vi "Write_Accelerometer_To_Read.vi"(8 "error in (no error)":errorcluster, 9 "Read ERD List":T2[](array[typedef]) {"ERD Number" format="%.0x"}, 10 "GEA Inputs":T1 {"Destination" format="%.0x"; "Source" format="%.0x"}, 11 ".NET Refnum in":refnum<k24>) -> (0 "error out":errorcluster, 3 ".NET Refnum out":refnum<k24>)   [LabVIEW 2016]
doc: "This VI checks to see if Accelerometer ERD is in Read ERD List. If so it write to Accelerometer ERD. Writing toi this ERD updates ERD with latest Accelerometer data, which allows it to be read back from ERD."
uses:
  Common/LabVIEW GEA2 Toolkit/LabVIEW_GEA2_Toolkit.lvlibp/type defs/ERD Read Data In.ctl
  Common/LabVIEW GEA2 Toolkit/LabVIEW_GEA2_Toolkit.lvlibp/type defs/Data Type.ctl
  Common/LabVIEW GEA2 Toolkit/LabVIEW_GEA2_Toolkit.lvlibp/type defs/Source_Destination.ctl
  C:/Automation/DLLs/PC Dot Net/GeaCommunication.dll
  Common/LabVIEW GEA2 Toolkit/LabVIEW_GEA2_Toolkit.lvlibp/type defs/ERD Write Data In.ctl
  Common/LabVIEW GEA2 Toolkit/LabVIEW_GEA2_Toolkit.lvlibp
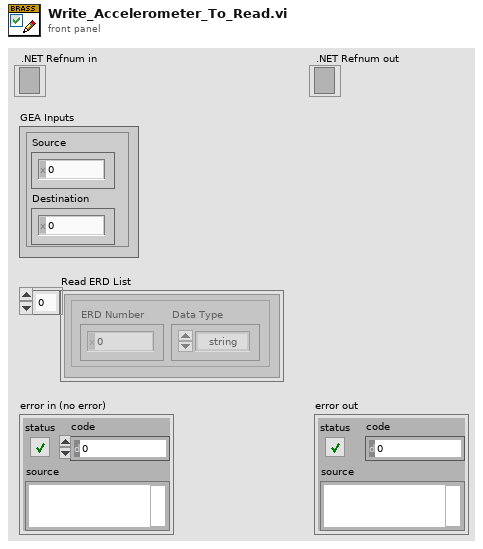
[diagram p1: front panel]
types:
  T1 = typedef "LabVIEW_GEA2_Toolkit.lvlibp/Source_Destination.ctl" = cluster{"Source":u8, "Destination":u8}
  T2 = typedef "LabVIEW_GEA2_Toolkit.lvlibp/ERD Read Data In.ctl" = cluster{"ERD Number":u16, "Data Type":T3}
  T3 = typedef "LabVIEW_GEA2_Toolkit.lvlibp/Data Type.ctl" = enum16{"string", "boolean", "uint8_t", "uint16_t", "uint32_t", "uint64_t", "int8_t", "int16_t", "int32_t", "int64_t"}
  T4 = typedef "LabVIEW_GEA2_Toolkit.lvlibp/ERD Write Data In.ctl" = cluster{"ERD Number":u16, "Data Type":T3, "Data":string}
  T5 = typedef "LabVIEW_GEA2_Toolkit.lvlibp/Data In.ctl" = cluster{"Source":u8, "Destination":u8, "Command":u8, "Message":string}
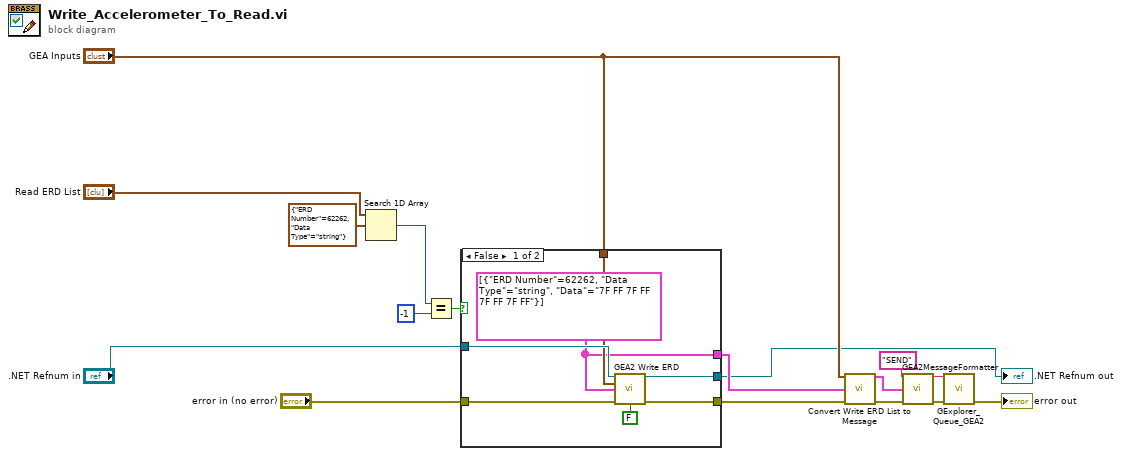
[diagram p0: block diagram]
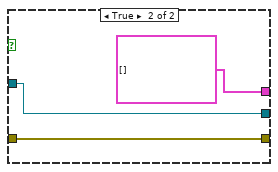
[diagram p2: hidden frame]
diagram:
  n1 = Search 1D Array(1D array="Read ERD List", element=T2 {"ERD Number"=62262, "Data Type"=enum."string"}) -> (index of element=w15:i32)  [unwired: 1 in]
  n2 = Equal?(x=w15, y=-1) -> (x = y?=w16:bool)
  n3 = case shown="False" w16 {
    tunnel: "error in (no error)" -> [w24 w26]
    tunnel: [w23 w26] -> w5
    tunnel: ".NET Refnum in" -> [w22 w27]
    tunnel: [w21 w27] -> w1
    tunnel: "GEA Inputs" -> [w20 _]
    tunnel: [w18 T4[] [] ("Write ERD List")] -> w2
    frame False {
      w18 = T4[] [{"ERD Number"=62262, "Data Type"=enum."string", "Data"="7F FF 7F FF 7F FF 7F FF"}] ("Write ERD List")
      n4 = call "GEA2 Write ERD.vi"("GEA2 Reference In"=w22, "GEA Inputs"=w20, "Write ERD List"=w18, "Error In"=w24, "Verify ERD Response?"=FALSE) -> ("GEA2 Reference Out"=w21:refnum<k24>, "Error Out"=w23:errorcluster)  [unwired: 8 in, 1 out]
    }
    frame True {
    }
  }
  ".NET Refnum out" <- w1
  n5 = call "Convert Write ERD List to Message.vi"("GEA Inputs"="GEA Inputs", "Write ERD List"=w2, "Error In"=w5) -> ("GEA Message"=w9:T5, "Error Out"=w10:errorcluster)  [unwired: 11 in]
  n6 = call "GEA2MessageFormatter.vi"("Prefix(Send/Recv)"="SEND", "GEA2 Data In"=w9, "Error In"=w10) -> ("Output String"=w8:string, "Error Out"=w7:errorcluster)  [unwired: 11 in]
  n7 = call "GExplorer_Queue_GEA2.vi"("Output String"=w8, "error in (no error)"=w7) -> ("error out"=→"error out":errorcluster)  [unwired: 13 in]
